vi "Configure 4 Wire Resistance.vi"(0 "VISA resource name":refnum<visa-resource-name>, 5 "Enable Low Power Resistance (T: Enable)":bool=TRUE, 7 "Enable Voltage Limited Resistance (F: Disable)":bool, 9 "Voltage Limit (1: 100 mV)":u16(ring)=100 items=["20 mV"=20, "100 mV"=100, "500 mV"=500], 11 "error in (no error)":errorcluster) -> (4 "VISA resource name out":refnum<visa-resource-name>, 15 "error out":errorcluster)   [LabVIEW 2021, in "Agilent 34420.lvlib"]
doc: "Configures the additional measurement modes available for 4 - wire resistance measurements."
uses:
  <instrlib>/Agilent 34420/Agilent 34420.lvlib
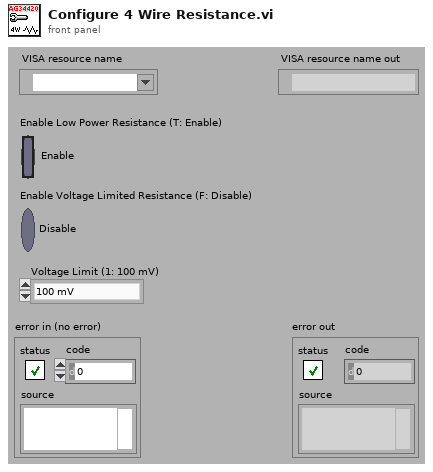
[diagram p1: front panel]
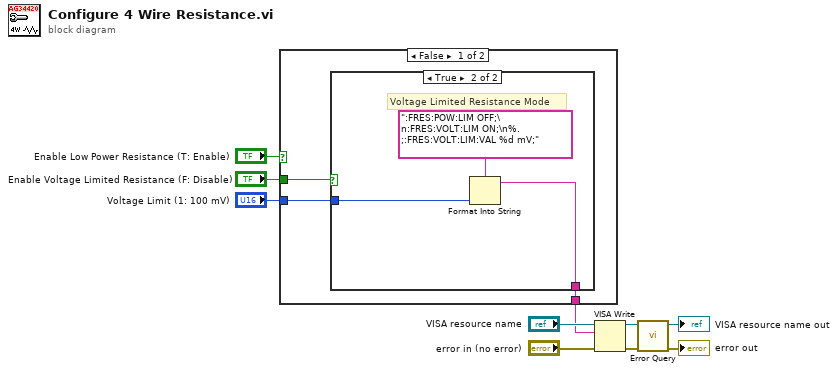
[diagram p0: block diagram]
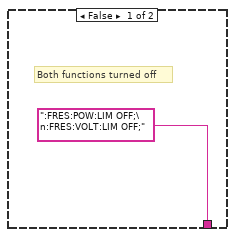
[diagram p2: hidden frame]
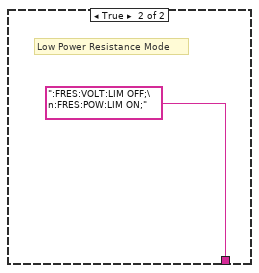
[diagram p3: hidden frame]
diagram:
  n1 = case shown="False" "Enable Low Power Resistance (T: Enable)" {
    tunnel: "Voltage Limit (1: 100 mV)" -> [w12 _]
    tunnel: "Enable Voltage Limited Resistance (F: Disable)" -> [w13 _]
    tunnel: [w11 ":FRES:VOLT:LIM OFF;\n:FRES:POW:LIM ON;"] -> w1
    frame False {
      n2 = case shown="True" w13 {
        tunnel: w12 -> [_ w15]
        tunnel: [":FRES:POW:LIM OFF;\n:FRES:VOLT:LIM OFF;" w16] -> w11
        frame False {
          # "Both functions turned off"
        }
        frame True {
          # "Voltage Limited Resistance Mode"
          n3 = Format Into String(format string=":FRES:POW:LIM OFF;\n:FRES:VOLT:LIM ON;\n%.;:FRES:VOLT:LIM:VAL %d mV;", w15) -> (resulting string=w16:string)  [unwired: 2 in, 1 out]
        }
      }
    }
    frame True {
      # "Low Power Resistance Mode"
    }
  }
  n4 = VISA Write(VISA resource name="VISA resource name", write buffer=w1, error in (no error)="error in (no error)") -> (VISA resource name out=w5:refnum<visa-resource-name>, error out=w4:errorcluster)  [unwired: 1 out]
  n5 = call <instrlib>:"Error Query.vi"("error in (no error)"=w4, "VISA resource name"=w5) -> ("error out"=→"error out":errorcluster, "VISA resource name out"=→"VISA resource name out":refnum<visa-resource-name>)  [unwired: 6 in, 2 out]
